vi "dram_clip_count.vi"(7 "reset":bool=TRUE, 11 "increment":bool=TRUE) -> (3 "count out":u32)   [LabVIEW 2014]
doc: "Upcount VI for DRAM memory. \nIncrements internal counter by 4 when increment is true. Resets internal counter to zero when reset is true.\nThe CLIP interfaces to DRAM read and write 4 consecutive memory addresses at once."
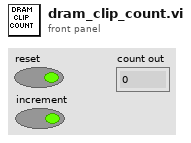
[diagram p1: front panel]
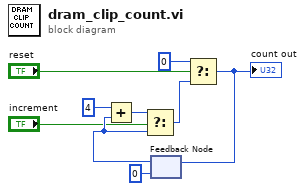
[diagram p0: block diagram]
diagram:
  n1 = feedback #1(u32 0) -> (w4:u32)
  n2 = Add(x=u32 4, y=w4) -> (x+y=w1:u32)
  n3 = Select(t=w1, s="increment", f=w4) -> (s? t:f=w7:u32)
  n4 = Select(t=u32 0, s="reset", f=w7) -> (s? t:f=w6:u32)
  "count out" <- w6
  n5 = feedback-in #1(w6) -> ()
